vi "dataset.get.vi"(8 "error in (no error)":errorcluster, 11 "target in":refnum<class "target.lvclass">) -> (0 "error out":errorcluster, 2 "datasources.lvlib:dataset.lvclass":refnum<class "dataset.lvclass">, 3 "target out":refnum<class "target.lvclass">)   [LabVIEW 2020, in "datasources.lvlib" / "target.lvclass"]
uses:
  target.lvclass
  dataset/dataset.lvclass
  target.lvclass/target.ctl
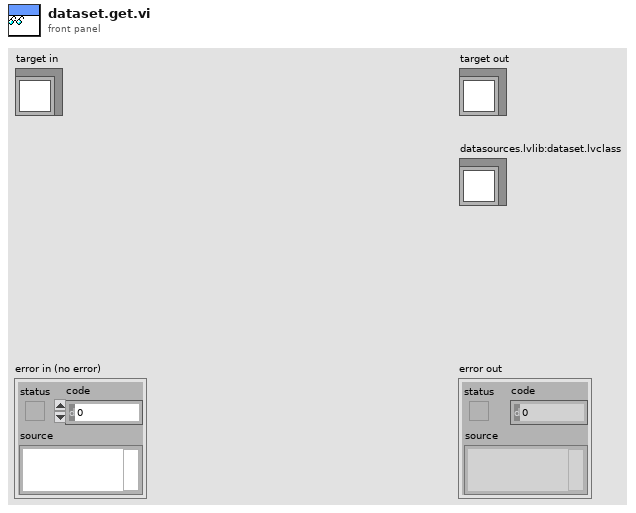
[diagram p1: front panel]
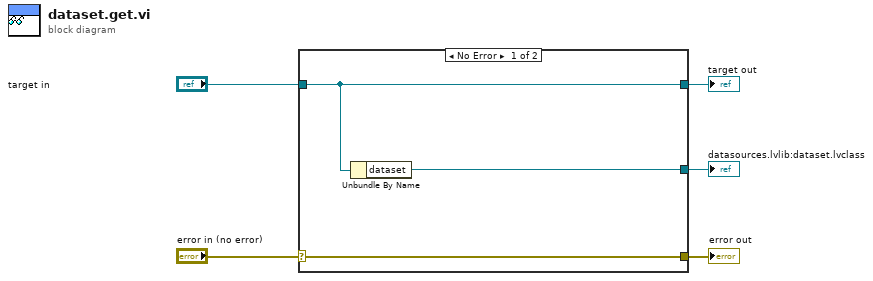
[diagram p0: block diagram]
diagram:
  n1 = case shown="No Error" "error in (no error)" {
    selector: "error in (no error)" -> [w8 w9]
    tunnel: [w8 w9] -> w4
    tunnel: [w7 w10] -> w2
    tunnel: "target in" -> [w7 w10]
    tunnel: [w6 _] -> w1
    frame No Error {
      n2 = Unbundle By Name(w7) -> ("dataset"=w6:refnum<class "dataset.lvclass">)
    }
    frame Error {
    }
  }
  "error out" <- w4
  "target out" <- w2
  "datasources.lvlib:dataset.lvclass" <- w1
